vi "TestExec.Distributed INI Config File Reader.vi"(8 "error in (no error)":errorcluster, 9 "Additional Config Section Names":string[](array[string])=["AdditionalConfig", "Station"], 10 "Initial Config File Path":path, 11 "Output Config Path":path) -> (0 "error out":errorcluster, 2 "Config File List":path[](array[path]), 3 "Output Config Path Dup":path)   [LabVIEW 2018]
uses:
  <vilib>/KATE/Status/Status Utils.lvlib
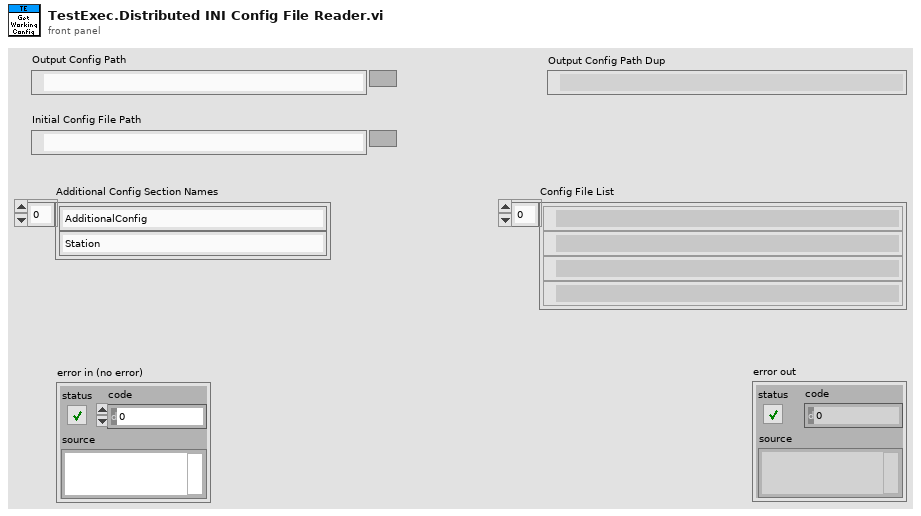
[diagram p1: front panel]
types:
  T1 = cluster{"Files":path[], "FileHist":path[], "AddSects":string[], "Output":path}
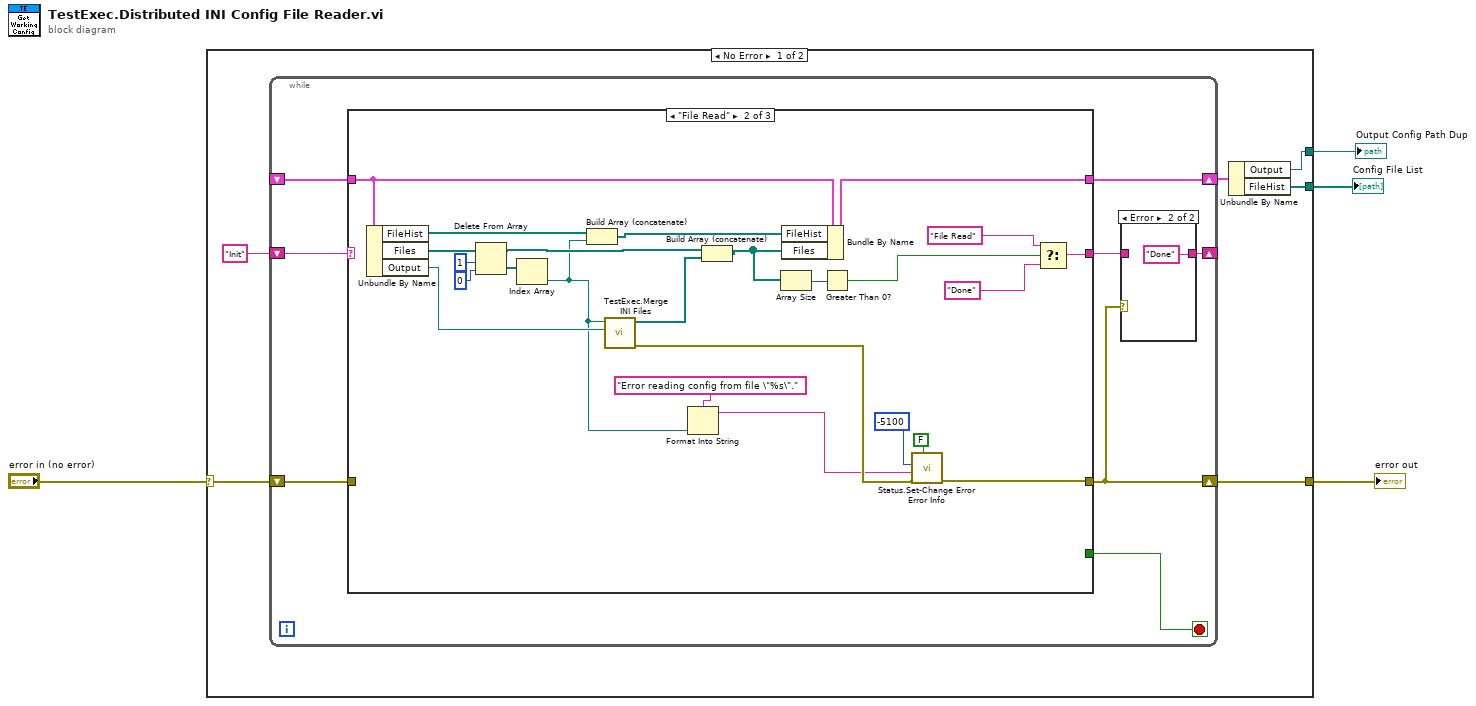
[diagram p0: block diagram]
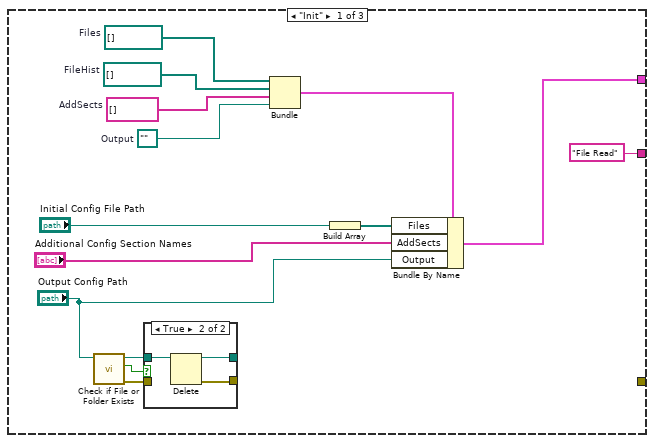
[diagram p3: hidden frame]
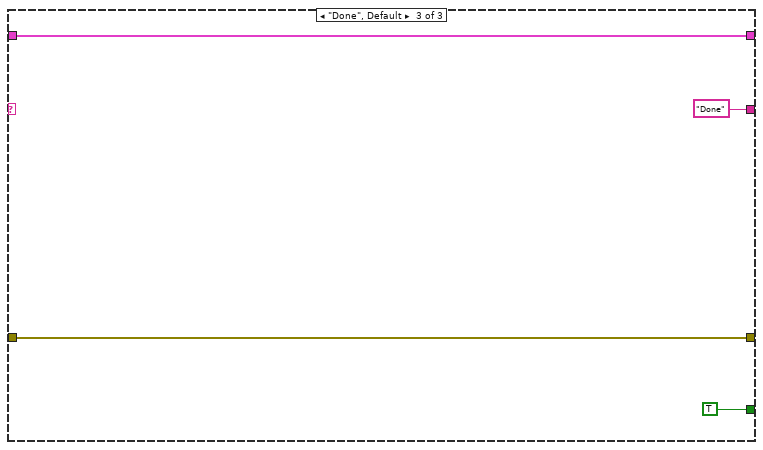
[diagram p5: hidden frame]
diagram:
  n1 = case shown="No Error" "error in (no error)" {
    selector: "error in (no error)" -> [w9 w67]
    tunnel: [w8 w67] -> w3
    tunnel: [w6 _] -> w2
    tunnel: [w5 _] -> w1
    frame No Error {
      n2 = while {
        shift-right: [w13] -> _
        shift-left: "Init" -> [w18]
        shift-right: [w16] -> w7
        shift-left: _ -> [w17]
        shift-right: [w11] -> w8
        shift-left: w9 -> [w12]
        stop <- w15 stop-if-true
        n3 = case shown="\"File Read\"" w18 {
          tunnel: w17 -> [_ w58 w64]
          tunnel: [w29 w57 w64] -> w16
          tunnel: ["File Read" w53 "Done"] -> w14
          tunnel: [_ _ TRUE] -> w15
          tunnel: w12 -> [_ _ w63]
          tunnel: [_ w42 w63] -> w11
          frame "Init" {
            w26 = path ""  # Output
            w27 = path[] []  # Files
            w33 = string[] []  # AddSects
            w34 = path[] []  # FileHist
            n4 = call <vilib>:"Check if File or Folder Exists.vi"("path"="Output Config Path") -> ("error out"=w23:errorcluster, "file or folder exists?"=w25:bool, "dup path"=w24:path)  [unwired: 8 in]
            n5 = case shown="True" w25 {
              tunnel: w24 -> [w35 w38]
              tunnel: w23 -> [_ _]
              tunnel: [w35 w37] -> _
              tunnel: [_ w36] -> _
              frame False {
              }
              frame True {
                n6 = Delete(path (use dialog)=w38) -> (deleted path=w37:path, error out=w36:errorcluster)  [unwired: 4 in, 1 out]
              }
            }
            n7 = Bundle("Files"=w27, "FileHist"=w34, "AddSects"=w33, "Output"=w26) -> (w32:T1)  [unwired: 1 in]
            n8 = Build Array("Initial Config File Path") -> (w21:path[])
            n9 = Bundle By Name(cluster=w32, "Files"=w21, "AddSects"="Additional Config Section Names", "Output"="Output Config Path") -> (w29:T1)
          }
          frame "File Read" {
            n10 = Unbundle By Name(w58) -> ("FileHist"=w56:path[], "Files"=w62:path[], "Output"=w49:path)
            n11 = Delete From Array(array=w62, length=1, index=0) -> (deleted portion=w59:path[], array with subset deleted=w48:path[])
            n12 = Index Array(array=w59) -> (element=w44:path)  [unwired: 1 in]
            n13 = Build Array (concatenate)(w56, w44) -> (w55:path[])
            n14 = call "TestExec.Merge INI Files.vi"("Dest File"=w49, "Source File"=w44) -> ("error out"=w43:errorcluster, "Files"=w47:path[])  [unwired: 8 in]
            n15 = Format Into String(format string="Error reading config from file \"%s\".", w44) -> (resulting string=w40:string)  [unwired: 2 in, 1 out]
            n16 = Build Array (concatenate)(w48, w47) -> (w46:path[])
            n17 = Array Size(array=w46) -> (size(s)=w54:i32)
            n18 = Bundle By Name(cluster=w58, "FileHist"=w55, "Files"=w46) -> (w57:T1)
            n19 = Greater Than 0?(x=w54) -> (x > 0?=w50:bool)
            n20 = call <vilib>:"Status.Set-Change Error Error Info.vi"("AppendOrigDesc"=FALSE, "Error In"=w43, "NewDesc"=w40, "NewCode"=-5100) -> ("Error Out"=w42:errorcluster)  [unwired: 7 in]
            n21 = Select(t="File Read", s=w50, f="Done") -> (s? t:f=w53:string)
          }
          frame "Done", Default {
          }
        }
        n22 = case shown="Error" w11 {
          tunnel: w14 -> [w19 _]
          tunnel: [w19 "Done"] -> w13
          frame No Error {
          }
          frame Error {
          }
        }
      }
      n23 = Unbundle By Name(w7) -> ("Output"=w5:path, "FileHist"=w6:path[])
    }
    frame Error {
    }
  }
  "Config File List" <- w2
  "Output Config Path Dup" <- w1
  "error out" <- w3
